vi "SubVI_CoEIndexRead.vi"() -> ()   [LabVIEW 2022 SP3, in "EtherCAT_Library.lvlib"]
doc: "This SubVI takes in a EtherCAT Device Address as input, in the format AMSNetID:EtherCATAddress, for example 127.0.0.0.1.1:1001\n\nThe Index and SubIndex inputs allow you to specify the CoE Index of the target to be read\n\nThe output is a cluster containing the Name, details and data from the CoE index."
uses:
  EtherCAT_Library.lvlib
panel:
  out "CoE Index Information":T1
  in  "Index":u16
  in  "Device address":string
  in  "SubIndex":u8
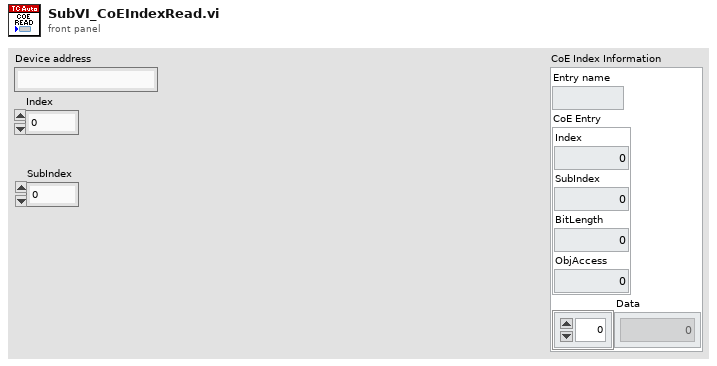
[diagram p1: front panel]
types:
  T1 = cluster{"Entry name":string, "CoE Entry":cluster{"Index":u16, "SubIndex":u8, "BitLength":u16, "ObjAccess":u16}, "Data":u8[]}
  T2 = cluster{"Index":u16, "SubIndex":u8, "BitLength":u16, "ObjAccess":u16}
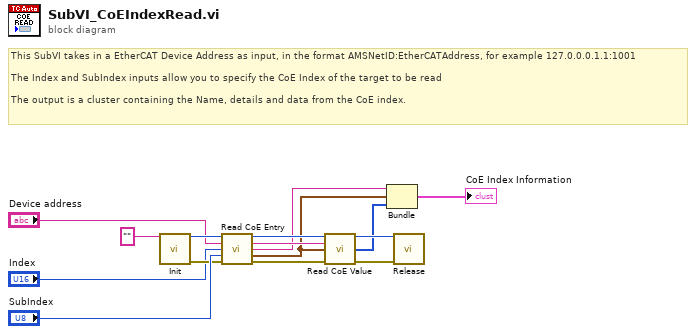
[diagram p0: block diagram]
diagram:
  # "This SubVI takes in a EtherCAT Device Address as input, in the format AMSNetID:EtherCATAddress, for example 127.0.0.0.1.1:1001\n\nThe Index and SubIndex inputs allow you to specify the CoE Index of the target to be read\n\nThe output is a cluster containing the Name, details and data from the CoE index."
  n1 = call <userlib>:"Init.vi"("XMLDescription"="") -> ("Handle"=w8:u32, "error out"=w7:errorcluster)  [unwired: 10 in, 3 out]
  n2 = call <userlib>:"Read CoE Entry.vi"("Handle"=w8, "Device address"="Device address", "Index"="Index", "SubIndex"="SubIndex", "error in (no error)"=w7) -> ("Handle"=w13:u32, "Device address"=w12:string, "Entry name"=w4:string, "CoE Entry"=w3:T2, "error out"=w11:errorcluster)  [unwired: 6 in]
  n3 = call <userlib>:"Read CoE Value.vi"("Handle"=w13, "Device address"=w12, "CoE entry"=w3, "error in (no error)"=w11) -> ("Handle"=w9:u32, "Data"=w2:u8[], "error out"=w10:errorcluster)  [unwired: 8 in, 1 out]
  n4 = Bundle("Entry name"=w4, "CoE Entry"=w3, "Data"=w2) -> (→"CoE Index Information":T1)  [unwired: 1 in]
  n5 = call <userlib>:"Release.vi"("Handle"=w9, "error in (no error)"=w10) -> ()  [unwired: 13 in, 1 out]
